vi "Write Abort Event and Time to Server.vi"(6 "Time Value (DBL)":dbl, 7 "Abort Event":string, 8 "error in (no error)":errorcluster, 11 "connection ID":refnum<k5>) -> (0 "error out":errorcluster, 3 "connection ID duplicate":refnum<k5>)   [LabVIEW 2010, in "Core SubVIs.lvlib"]
uses:
  Core SubVIs.lvlib
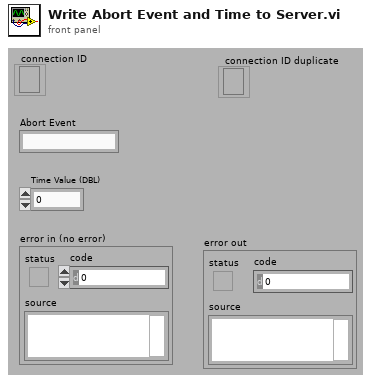
[diagram p1: front panel]
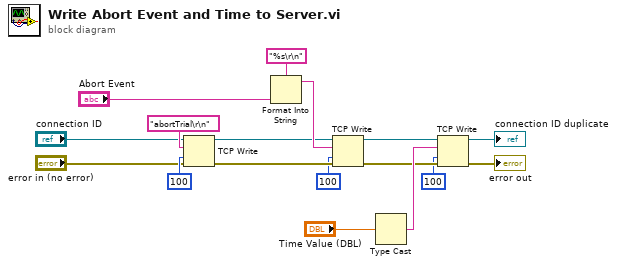
[diagram p0: block diagram]
diagram:
  n1 = TCP Write(connection ID="connection ID", data in="abortTrial\r\n", error in (no error)="error in (no error)", 9:100 ("timeout ms (25000)")) -> (connection ID out=w6:refnum<k5>, error out=w7:errorcluster)  [unwired: 1 out]
  n2 = Format Into String(format string="%s\r\n" ("data in"), "Abort Event") -> (resulting string=w17:string)  [unwired: 2 in, 1 out]
  n3 = TCP Write(connection ID=w6, data in=w17, error in (no error)=w7, 9:100 ("timeout ms (25000)")) -> (connection ID out=w9:refnum<k5>, error out=w10:errorcluster)  [unwired: 1 out]
  n4 = Type Cast(x="Time Value (DBL)") -> (*(type *) &x=w12:string)  [unwired: 1 in]
  n5 = TCP Write(connection ID=w9, data in=w12, error in (no error)=w10, 9:100 ("timeout ms (25000)")) -> (connection ID out=→"connection ID duplicate":refnum<k5>, error out=→"error out":errorcluster)  [unwired: 1 out]
